vi "LeCroy_Control_Enumerator.vi"(8 "Time/Div (S) Ref":refnum<vi>, 9 "Voltage (V/div) Ref":refnum<vi>, 10 "Sampling Rate (MHz) Ref":refnum<vi>) -> (1 "Voltage (V/div)":cluster{"String":string, "Value":dbl}[](array[cluster]), 2 "Time/div (us)":cluster{"String":string, "Value":dbl}[](array[cluster]), 3 "Sample Rate (MHz)":cluster{"String":string, "Value":dbl}[](array[cluster]))   [LabVIEW 2022 SP3]
uses:
  <vilib>/Utility/miscctls.llb/LVStringsAndValuesArrayTypeDef_U16.ctl
  -DigitizerRoutines/DigitizerGlobals.vi
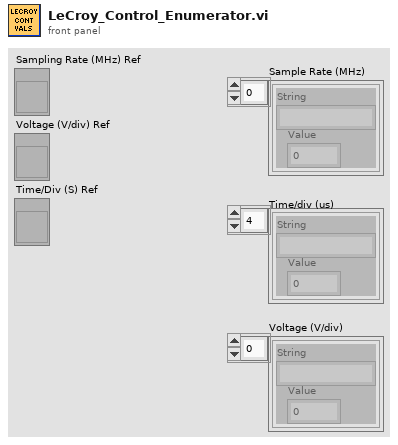
[diagram p1: front panel]
types:
  T1 = typedef "DigitizerSettings.ctl" = cluster{"Digitizer delay (us) ":dbl, "rf points per line":i32, "lines per plane":i32, "Samp Rate (Hz)":dbl, "Additional dig delay (us)":dbl, "Voltage Scale":dbl, "Pre-Looks":i32, "Offset delay (us)":dbl, "bits A/D":i8, "Avg Num":i32, "DigTimeOut":sgl, "Rel Dig Delay":sgl, "Dig Ch":i32, "LeCroyCluster":cluster{"LeCroy Channels":bool[], "LC read pt offset":dbl, "Sweep Avg":bool}, "Main Digitizer":T2, "Dig Config":T3, "Digitizer ID Cluster":T4, "Trigger Settings":cluster{"Trig Source":u16, "Trig Coupling":u16, "Trig Slope":u16, "Level (mV)":dbl}, "Bulk Acq":bool, "Bulk Start Indexes":i32[], "Data Ref RF":refnum<data-value>, "NI ID/Channel":cluster{"NI ID":refnum<k15>, "NI CH":i32}[], "Total Dig CH":i32, "Xtra Ann Trig delay (us)":dbl, "Fix Z Delay?":bool, "One Way Transmission?":bool, "Data Ref Log":refnum<data-value>}
  T2 = typedef "Digitizer.ctl" = enum16{"Acqiris Digitizer", "NI Digitizer", "LeCroy", "GaGe", "AlazarTech", "No Digitizer", "Teledyne"}
  T3 = typedef "DigConfig.ctl" = enum16{"Single channel", "2 Chans w/ 2 Acqiris", "2 Chans w/ 1 Acqiris", "5-CH Pulser New", "5-CH pulser w/ ann array", "5-pass style ann array", "Empty"}
  T4 = typedef "DigitizerID.ctl" = cluster{"Acqiris/Alazar/SP ID":u32[], "NI Instr Handles":refnum<k15>[], "LeCroy VISA":refnum<visa-resource-name>, "GaGe Handle":cluster{"Handle":u32, "Sample size":u32, "Resolution":i32, "Offset":i32, "Channels":u32, "Boards":u32}, "ATS Ref":string, "Acqiris Address":string[], "ADQRef":refnum<k24>, "adq_cu_ptr":refnum<k24>}
  T5 = typedef "LVStringsAndValuesArrayTypeDef_U16.ctl" = cluster{"String":string, "Value":u16}[]
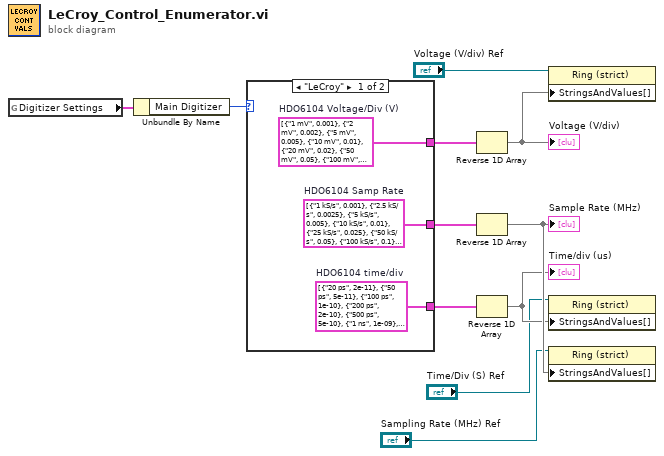
[diagram p0: block diagram]
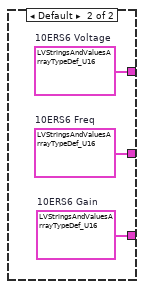
[diagram p2: hidden frame]
diagram:
  n1 = global read "DigitizerGlobals.vi" "Digitizer Settings"() -> (w4:T1)
  n2 = Unbundle By Name(w4) -> ("Main Digitizer"=w3:T2)
  n3 = case shown="\"LeCroy\"" w3 {
    tunnel: [w12 w15] -> w8
    tunnel: [w13 w16] -> w10
    tunnel: [w14 w17] -> w9
    frame "LeCroy" {
      w14 = cluster{"String":string, dbl}[] [{"String"="1 mV", 0.001}, {"String"="2 mV", 0.002}, {"String"="5 mV", 0.005}, {"String"="10 mV", 0.01}, {"String"="20 mV", 0.02}, {"String"="50 mV", 0.05}, {"String"="100 mV", 0.1}, {"String"="200 mV", 0.2}, {"String"="500 mV", 0.5}, {"String"="1 V", 1.0}]  # HDO6104 Voltage/Div (V)
      w13 = cluster{"String":string, dbl}[] [{"String"="20 ps", 2e-11}, {"String"="50 ps", 5e-11}, {"String"="100 ps", 1e-10}, {"String"="200 ps", 2e-10}, {"String"="500 ps", 5e-10}, {"String"="1 ns", 1e-09}, {"String"="2 ns", 2e-09}, {"String"="5 ns", 5e-09}, {"String"="10 ns", 1e-08}, {"String"="20 ns", 2e-08}, {"String"="50 ns", 5e-08}, {"String"="100 ns", 1e-07}, {"String"="200 ns", 2e-07}, {"String"="500 ns", 5e-07}, {"String"="1 us", 1e-06}, {"String"="2 us", 2e-06}, {"String"="5 us", 5e-06}, {"String"="10 us", 1e-05}, {"String"="20 us", 2e-05}, {"String"="50 us", 5e-05}, {"String"="100 us", 0.0001}, {"String"="200 us", 0.0002}, {"String"="500 us", 0.0005}, {"String"="1 ms", 0.001}, {"String"="2 ms", 0.002}, {"String"="5 ms", 0.005}, {"String"="10 ms", 0.01}, {"String"="20 ms", 0.02}, {"String"="50 ms", 0.05}, {"String"=" 100 ms", 0.1}, {"String"="200 ms", 0.2}, {"String"="500 ms", 0.5}, {"String"="1 s", 1.0}, {"String"="2 s", 2.0}, {"String"="5 s", 5.0}, {"String"="10 s", 10.0}, {"String"="20 s", 20.0}, {"String"=" 50 s", 50.0}, {"String"="100 s", 100.0}, {"String"=" 200 s", 200.0}, {"String"=" 500 s", 500.0}, {"String"="1 ks", 1000.0}, {"String"="2 ks", 2000.0}, {"String"="5 ks", 5000.0}]  # HDO6104 time/div
      w12 = cluster{"String":string, dbl}[] [{"String"="1 kS/s", 0.001}, {"String"="2.5 kS/s", 0.0025}, {"String"="5 kS/s", 0.005}, {"String"="10 kS/s", 0.01}, {"String"="25 kS/s", 0.025}, {"String"="50 kS/s", 0.05}, {"String"="100 kS/s", 0.1}, {"String"="250 kS/s", 0.25}, {"String"="500 kS/s", 0.5}, {"String"="1 MS/s", 1.0}, {"String"="2.5 MS/s", 2.5}, {"String"="5 MS/s", 5.0}, {"String"="10 MS/s", 10.0}, {"String"="25 MS/s", 25.0}, {"String"="50 MS/s", 50.0}, {"String"="100 MS/s", 100.0}, {"String"="250 MS/s", 250.0}, {"String"="500 MS/s", 500.0}, {"String"="1.25 GS/s", 1250.0}, {"String"="2.5 GS/s", 2500.0}, {"String"="5 GS/s", 5000.0}, {"String"="10 GS/s", 10000.0}, {"String"="20 GS/s", 20000.0}, {"String"="40 GS/s", 40000.0}]  # HDO6104 Samp Rate
    }
    frame Default {
      w17 = T5 [{"String"="0", "Value"=0}, {"String"="5", "Value"=5}, {"String"="10", "Value"=10}, {"String"="15", "Value"=15}, {"String"="20", "Value"=20}, {"String"="25", "Value"=25}, {"String"="30", "Value"=30}, {"String"="35", "Value"=35}, {"String"="40", "Value"=40}, {"String"="45", "Value"=45}, {"String"="50", "Value"=50}, {"String"="55", "Value"=55}, {"String"="60", "Value"=60}, {"String"="65", "Value"=65}, {"String"="70", "Value"=70}, {"String"="75", "Value"=75}, {"String"="80", "Value"=80}, {"String"="85", "Value"=85}, {"String"="90", "Value"=90}, {"String"="95", "Value"=95}, {"String"="100", "Value"=100}]  # 10ERS6 Voltage
      w16 = T5 [{"String"="22", "Value"=22}, {"String"="25", "Value"=25}, {"String"="28", "Value"=28}, {"String"="31", "Value"=31}, {"String"="34", "Value"=34}, {"String"="37", "Value"=37}, {"String"="40", "Value"=40}, {"String"="43", "Value"=43}, {"String"="46", "Value"=46}, {"String"="49", "Value"=49}, {"String"="52", "Value"=52}, {"String"="55", "Value"=55}, {"String"="58", "Value"=58}, {"String"="61", "Value"=61}, {"String"="64", "Value"=64}, {"String"="67", "Value"=67}]  # 10ERS6 Gain
      w15 = T5 [{"String"="4", "Value"=4}, {"String"="5", "Value"=5}, {"String"="6", "Value"=6}, {"String"="8", "Value"=8}, {"String"="10", "Value"=10}, {"String"="12", "Value"=12}, {"String"="14", "Value"=14}, {"String"="16", "Value"=16}, {"String"="18", "Value"=18}, {"String"="20", "Value"=20}, {"String"="25", "Value"=25}, {"String"="30", "Value"=30}, {"String"="35", "Value"=35}, {"String"="40", "Value"=40}, {"String"="45", "Value"=45}, {"String"="50", "Value"=50}]  # 10ERS6 Freq
    }
  }
  n4 = Reverse 1D Array(array=w9) -> (reversed array=w6:cluster{"String":string, "Value":dbl}[])
  "Voltage (V/div)" <- w6
  n5 = Reverse 1D Array(array=w8) -> (reversed array=w7:cluster{"String":string, "Value":dbl}[])
  "Sample Rate (MHz)" <- w7
  n6 = Reverse 1D Array(array=w10) -> (reversed array=w5:cluster{"String":string, "Value":dbl}[])
  "Time/div (us)" <- w5
  n7 = property class="Ring (strict)"(reference="Voltage (V/div) Ref", "StringsAndValues[]"=w6) -> ()  [unwired: 1 in, 2 out]
  n8 = property class="Ring (strict)"(reference="Time/Div (S) Ref", "StringsAndValues[]"=w5) -> ()  [unwired: 1 in, 2 out]
  n9 = property class="Ring (strict)"(reference="Sampling Rate (MHz) Ref", "StringsAndValues[]"=w7) -> ()  [unwired: 1 in, 2 out]
